vi "Voltage - Timed Loop.vi"() -> ()   [LabVIEW 2022 SP3]
doc: "This example demonstrates how to continuously acquire voltage measurements from a DAQmx device using hardware timed, single point reads using a timed loop structure. The timed loop is controlled by the sample clock of the DAQ device. The device will read data on each tick of the sample clock. If an additional sample clock tick occurs before the current data point is read from the device or if the timed loop does not receive any sample clock ticks, a dialog will indicate that this has happened. \n\nHardware Timed Single Point acquisition works best when using a deterministic operating system (such as LabVIEW Real-Time). Because of the less deterministic nature of general purpose operating systems (such as Microsoft Windows), the software loop will not always take the exact same amount of time to execute, and this may lead to the occasional missed sample clock. \n\nFor instructions on how to connect your signals to the DAQ device, refer to your device documentation."
uses:
  <vilib>/Utility/error.llb/DialogType.ctl
  <vilib>/Platform/TimedLoop/XDataNode/timing_clust.ctl
  <vilib>/Platform/TimedLoop/XDataNode/nitl_modes.ctl
  <vilib>/Platform/TimedLoop/XDataNode/wakeup.ctl
  <vilib>/DAQmx/read.llb/DAQmx Read (Analog 1D DBL NChan 1Samp).vi
  <vilib>/DAQmx/create/channels.llb/DAQmx Create Channel (AI-Voltage-Basic).vi
  <vilib>/DAQmx/configure/timing.llb/DAQmx Timing (Sample Clock).vi
  <vilib>/DAQmx/create/timing.llb/DAQmx Create Timing Source (Signal From Task).vi
  <vilib>/DAQmx/miscellaneous.llb/DAQmx Fill In Error Info.vi
  <vilib>/Platform/TimedLoop/XDataNode/XDataNode.xnode
  <resource>/objmgr/daqmx.rc
  <vilib>/Platform/TimedLoop/XDataNode/XDNodeRunTimeDep.lvlib
panel:
  in  "Stop":bool
  out "Waveform Chart":dbl[](graph)
  in  "Sample Rate":dbl=100.0
  in  "Sample Clock Source":tag="OnboardClock"
  in  "Terminal Configuration":i32(ring)=-1 items=["default"=-1, "RSE"=10083, "NRSE"=10078, "Differential"=10106, "Pseudodifferential"=12529]
  in  "Max Voltage":dbl=5.0
  in  "Min Voltage":dbl=-5.0
  in  "Physical Channel":tag="Dev1/ai0"
  out "Actual Sample Rate":dbl=100.0 format="%0.2f"
  # "Channel Settings"
  # "Acquired Data"
  # "Timing Settings"
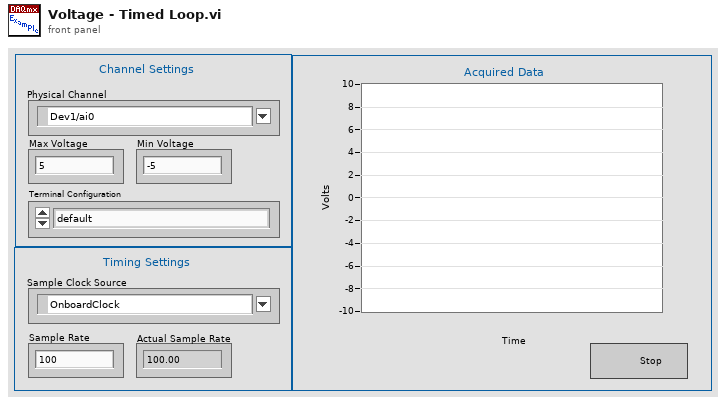
[diagram p1: front panel]
types:
  T1 = typedef "DialogType.ctl" = u16
  T2 = typedef "XDNodeRunTimeDep.lvlib/timing_clust.ctl" = cluster{"Expected End [f-1]":u64, "Actual End [f-1]":u64, "Finished Late? [f-1]":bool, "Expected End [i-1]":u64, "Actual End [i-1]":u64, "Finished Late? [i-1]":bool, "Expected Start [i]":u64, "Actual Start [i]":u64, "Expected Start [f]":u64, "Actual Start [f]":u64, "Source Name":string, "Structure Name":string, "Period":i64, "Deadline":i64, "Offset":i64, "Start":i64, "Priority":i32, "Timeout":i32, "Mode":T3, "Wakeup Reason":T4, "Error":errorcluster, "Source Type":string, "Secondary Source Type":string, "Global End Time":u64, "Global Start Time":u64, "Frame Duration":u64, "Iteration Duration":u64, "Assigned CPU":i32, "I/O Scan Engine Mode":u32}
  T3 = typedef "XDNodeRunTimeDep.lvlib/nitl_modes.ctl" = enum32{"No Change", "Process missed periods, maintain original phase", "Discard missed periods, maintain original phase", "Process missed periods, ignore original phase", "Discard missed periods, ignore original phase"}
  T4 = typedef "XDNodeRunTimeDep.lvlib/wakeup.ctl" = enum32{"Normal", "Aborted", "Asynchronous wakeup", "Timing source error", "Timed loop error", "Timeout"}
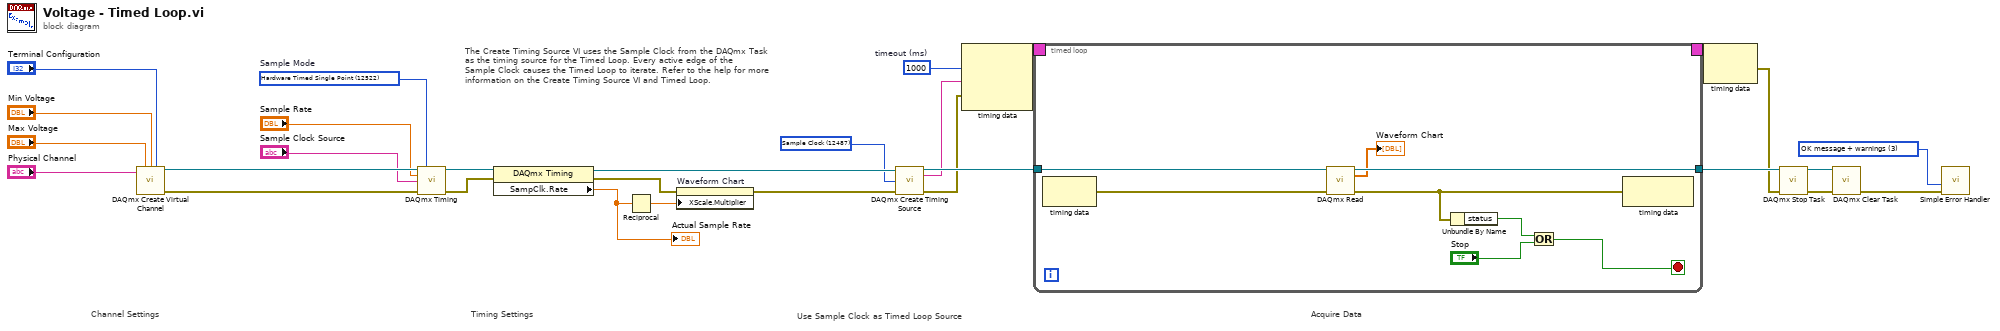
[diagram p0: block diagram]
diagram:
  w3 = 1000  # timeout (ms)
  w4 = 12487 items=["Sample Complete Event"=12530, "Counter Output Event"=12494, "Change Detection Event"=12511, "Sample Clock"=12487] ("signal")
  w12 = T1 3 items=["no dialog", "OK message", "continue or stop message", "OK message + warnings", "continue/stop + warnings"] ("type of dialog (OK msg:1)")
  w27 = 12522 items=["Finite Samples"=10178, "Continuous Samples"=10123, "Hardware Timed Single Point"=12522]  # Sample Mode
  # "The Create Timing Source VI uses the Sample Clock from the DAQmx Task\nas the timing source for the Timed Loop. Every active edge of the\nSample Clock causes the Timed Loop to iterate. Refer to the help for more\ninformation on the Create Timing Source VI and Timed Loop."
  # "Use Sample Clock as Timed Loop Source"
  # "Acquire Data"
  # "Timing Settings"
  # "Channel Settings"
  n1 = call-poly <vilib>:"DAQmx Create Virtual Channel.vi"("maximum value"="Max Voltage", "minimum value"="Min Voltage", "input terminal configuration"="Terminal Configuration", "physical channels"="Physical Channel") -> ("task out"=w25:refnum<k21>, "error out"=w26:errorcluster)  [unwired: 10 in]
  n2 = call-poly <vilib>:"DAQmx Timing.vi"("task/channels in"=w25, "sample mode"=w27, "rate"="Sample Rate", "source"="Sample Clock Source", "error in"=w26) -> ("task out"=w29:refnum<k21>, "error out"=w28:errorcluster)  [unwired: 9 in]
  n3 = property class="DAQmx Timing"(reference=w29, error in=w28) -> (reference out=w13:refnum<k21>, error out=w8:errorcluster, "SampClk.Rate"=w10:dbl)
  "Actual Sample Rate" <- w10
  n4 = Reciprocal(x=w10) -> (1/x=w11:dbl)
  n5 = property on="Waveform Chart" class="WFChart (strict)"(error in=w8, "XScale.Multiplier"=w11) -> (error out=w9:errorcluster)  [unwired: 1 in, 1 out]
  n6 = call-poly <vilib>:"DAQmx Create Timing Source.vi"("task/channels in"=w13, "signal"=w4, "error in"=w9) -> ("task out"=w24:refnum<k21>, "timing source out"=w5:string, "error out"=w2:errorcluster)  [unwired: 10 in]
  n7 = node-c288(w3, w5, w2) -> (w7:T2)
  n8 = timed-loop {
    timing: w7 -> [_]
    timing-out: [_] -> w6
    tunnel: w24 -> [w37]
    tunnel: [w36] -> w16
    stop <- w35 stop-if-true
    n9 = node-c288() -> (w34:errorcluster)  [unwired: 1 in]
    n10 = call-poly <vilib>:"DAQmx Read.vi"("task/channels in"=w37, "error in"=w34) -> ("task out"=w36:refnum<k21>, "data"=→"Waveform Chart":dbl[], "error out"=w33:errorcluster)  [unwired: 11 in]
    n11 = Unbundle By Name(w33) -> ("status"=w30:bool)
    n12 = Or(x=w30, y="Stop") -> (x .or. y?=w35:bool)
    n13 = node-c288(w33) -> ()  [unwired: 1 out]
  }
  n14 = node-c288(w6) -> (w1:errorcluster)
  n15 = call <vilib>:"DAQmx Stop Task.vi"("task/channels in"=w16, "error in"=w1) -> ("task out"=w14:refnum<k21>, "error out"=w15:errorcluster)  [unwired: 12 in]
  n16 = call <vilib>:"DAQmx Clear Task.vi"("task in"=w14, "error in"=w15) -> ("error out"=w23:errorcluster)  [unwired: 13 in]
  n17 = call <vilib>:"Simple Error Handler.vi"("type of dialog (OK msg:1)"=w12, "error in (no error)"=w23) -> ()  [unwired: 3 in, 5 out]
